vi "thermal measure Volt&SA.vi"(0 "meas_setting":T3={"measSetId"=6949, "measSetComments"="Orchid", "probeId"=141.0, "beamstyleIndex"=0, "txFrequencyHz"=3636400.0, "focusRangeCm"=8.0, "maxTxVoltageVolt"=100.0, "ceilTxVoltageVolt"=80.0, "profTxVoltageVolt"=62.0, "totalVoltagePt"=20, "numMeasVoltage"=12, "numTxElements"=118, "txpgWaveformStyle"=2, "numTxCycles"=4.0, "elevAperIndex"=0, "zStartDistCm"=1.5, "zMeasNum"=80, "IsTxAperModulationEn"=0, "DTxFreqIndex"=0, "VTxIndex"=0, "IsCPAEn"=0, "SysPulserSelA"=0, "TxPulseRleA"=""} {"zStartDistCm" format="%.2f"; "numTxCycles" format="%.1f"; "profTxVoltageVolt" format="%#_1g"; "ceilTxVoltageVolt" format="%.2f"; "maxTxVoltageVolt" format="%.2f"; "focusRangeCm" format="%.1f"; "txFrequencyHz" format="%.2f"}, 1 "PRF":dbl format="%.2f", 2 "CW":bool, 3 "measSetNum":i16, 4 "RoiLaterMin":dbl format="%.2f", 5 "TCP from Orchid in":refnum<k5>, 6 "RoiLateralSpan":dbl format="%.2f", 7 "Database":T4={"DB name"="zaop", "UID"="sel00752", "password"="rhkdwo7978"}, 8 "Measurement Type":enum32{"Volt", "SA"}(radio), 9 "tcp time out":dbl format="%.2f", 11 "voltage":dbl format="%.2f", 12 "Comment(SN)":string, 13 "Entire_element":u16, 14 "NumTxElement":i16) -> (10 "Command\nVerify":bool, 15 "Error(Volt & PRF)":bool)   [LabVIEW 2016]
uses:
  type def/Database.ctl
  type def/measSetting.ctl
  user/GrobaLimitVoltage.vi
  Thermal_type.vi
  <vilib>/Instr/_visa.llb/VISA Configure Serial Port (Instr).vi
  Instance          16 28Saved   thermal measure main .vi
  Instance          20 28Saved   thermal measure main .vi
panel:
  out "error out 4":errorcluster
  out "error out 3":errorcluster
  in  "취소 버튼":bool
  out "Measurement Time":enum32{"5min", "30min"}(radio)
  out "Voltage":dbl
  out "PRF":dbl
  out "right scanrange":dbl(slide) scale=0.0..30.1
  out "left scanrange":dbl(slide) max=3.0
  out "right aperture":u8(slide) scale=0.0..64.0
  out "left aperture":u8(slide) max=3
  out "경과시간(S)":string caption="경과 시간 텍스트"
  out "TempRise":dbl format="%.2f"
  out "Probe":dbl format="%.2f"
  out "Ambient":dbl format="%.2f"
  out "Waveform Chart":cluster{dbl, dbl}(graph)
  out "Actual PRF":dbl
  out "경과시간":dbl caption="경과 시간(초)" format="%#.1g"
  out "Ambient":dbl
  out "Transducer":dbl
  out "error out 2":errorcluster
  out "Input PRF":dbl format="%.2f"
  out "Current Voltage":dbl format="%.2f"
  out "Output Limit Voltage":i16
  out "Start Time":string="7/29/2002  5:00 PM"
  out "Finish Time":string="7/29/2002  5:00 PM"
  out "meas_temparature_output":T1 {"scanRange" format="%.2f"; "txpgWaveformStyle" format="%.2f"; "temperatureC" format="%.2f"; "pulseVoltage" format="%.2f"; "roomTempC" format="%.2f"; "probeId" format="%#.2f"}
  in  "stop 3":bool
  out "error out2":errorcluster
  in  "meas_temparature_result":T2={"probeId"=10.0, "comments"="4C1 WCS", "tempSSId"=2, "measDate"="", "measSetNum"=1, "roomTempC"=0.0, "pulseVoltage"=80.0, "temperatureC"=0.0, "numTxCycles"=3.0, "numTxElements"=22, "txFrequencyHz"=3636400, "elevAperIndex"=0, "isTxAperModulationEn"=0, "txpgWaveformStyle"=0.0, "pulseRepetRate"=610.0, "scanRange"=0.0, "tempSetId"=0, "IsSCW"=0, "VTxIndex"=0} {"temperatureC" format="%.2f"; "scanRange" format="%.2f"; "pulseRepetRate" format="%.6f"; "txpgWaveformStyle" format="%.3f"; "roomTempC" format="%.2f"; "numTxCycles" format="%#_1f"; "probeId" format="%#.2f"}
  in  "floating-point type conversion 2":string[][](table)=[["extended", "5", "12"], ["double", "5", "9"], ["single", "5", "5"]]
  out "Result":string
  in  "file path":path=path "C:/temp log data/TempResultData"
  out "error out":errorcluster
  # "Temperature Measurement"
  # "Cooling"
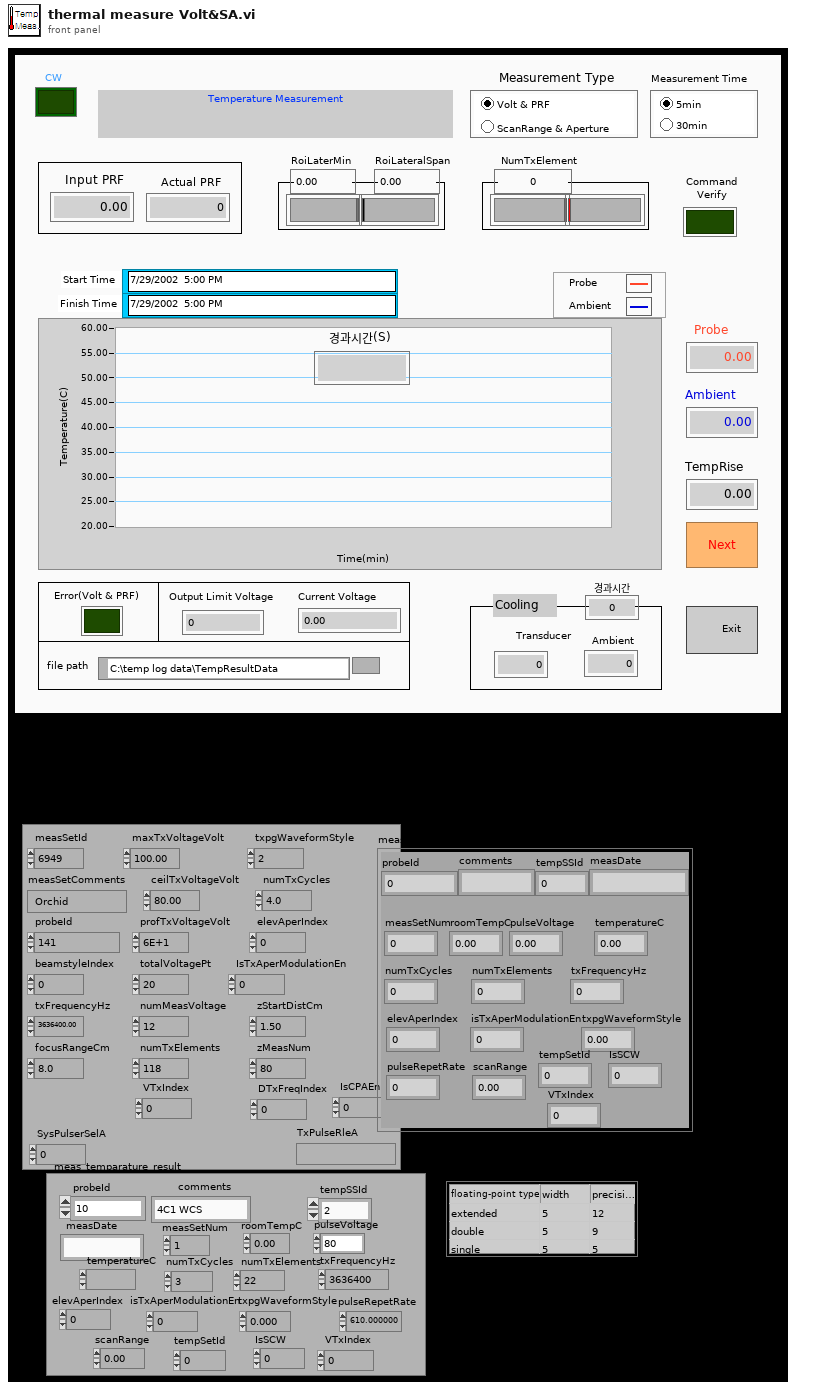
[diagram p1: front panel]
types:
  T1 = cluster{"probeId":sgl, "comments":string, "tempSSId":i16, "measDate":string, "measSetNum":i16, "roomTempC":sgl, "pulseVoltage":dbl, "temperatureC":ext, "numTxCycles":dbl, "numTxElements":i16, "txFrequencyHz":i32, "elevAperIndex":i16, "isTxAperModulationEn":i16, "txpgWaveformStyle":sgl, "pulseRepetRate":i32, "scanRange":dbl, "tempSetId":i16, "IsSCW":i16, "VTxIndex":i16}
  T2 = cluster{"probeId":sgl, "comments":string, "tempSSId":i16, "measDate":string, "measSetNum":i16, "roomTempC":sgl, "pulseVoltage":dbl, "temperatureC":ext, "numTxCycles":dbl, "numTxElements":i16, "txFrequencyHz":i32, "elevAperIndex":i16, "isTxAperModulationEn":i16, "txpgWaveformStyle":sgl, "pulseRepetRate":dbl, "scanRange":dbl, "tempSetId":i16, "IsSCW":i16, "VTxIndex":i8}
  T3 = typedef "measSetting.ctl" = cluster{"measSetId":i32, "measSetComments":string, "probeId":sgl, "beamstyleIndex":i16, "txFrequencyHz":sgl, "focusRangeCm":sgl, "maxTxVoltageVolt":sgl, "ceilTxVoltageVolt":sgl, "profTxVoltageVolt":dbl, "totalVoltagePt":i8, "numMeasVoltage":i8, "numTxElements":i16, "txpgWaveformStyle":i8, "numTxCycles":sgl, "elevAperIndex":i8, "zStartDistCm":sgl, "zMeasNum":i8, "IsTxAperModulationEn":i8, "DTxFreqIndex":i16, "VTxIndex":i8, "IsCPAEn":i16, "SysPulserSelA":i16, "TxPulseRleA":string}
  T4 = typedef "Database.ctl" = cluster{"DB name":string, "UID":string, "password":string}
  T5 = enum16{"open", "open or create", "create or replace", "create", "open (read only)"}
  T6 = cluster{"Output probe":dbl, "Output ambient":dbl}
  T7 = cluster{"status":bool, "code":i32, "text":string}
  T8 = typedef "Connection - Recordset reference.ctl" = cluster{"Connection":refnum<k7>, "Recordset":refnum<k7>}
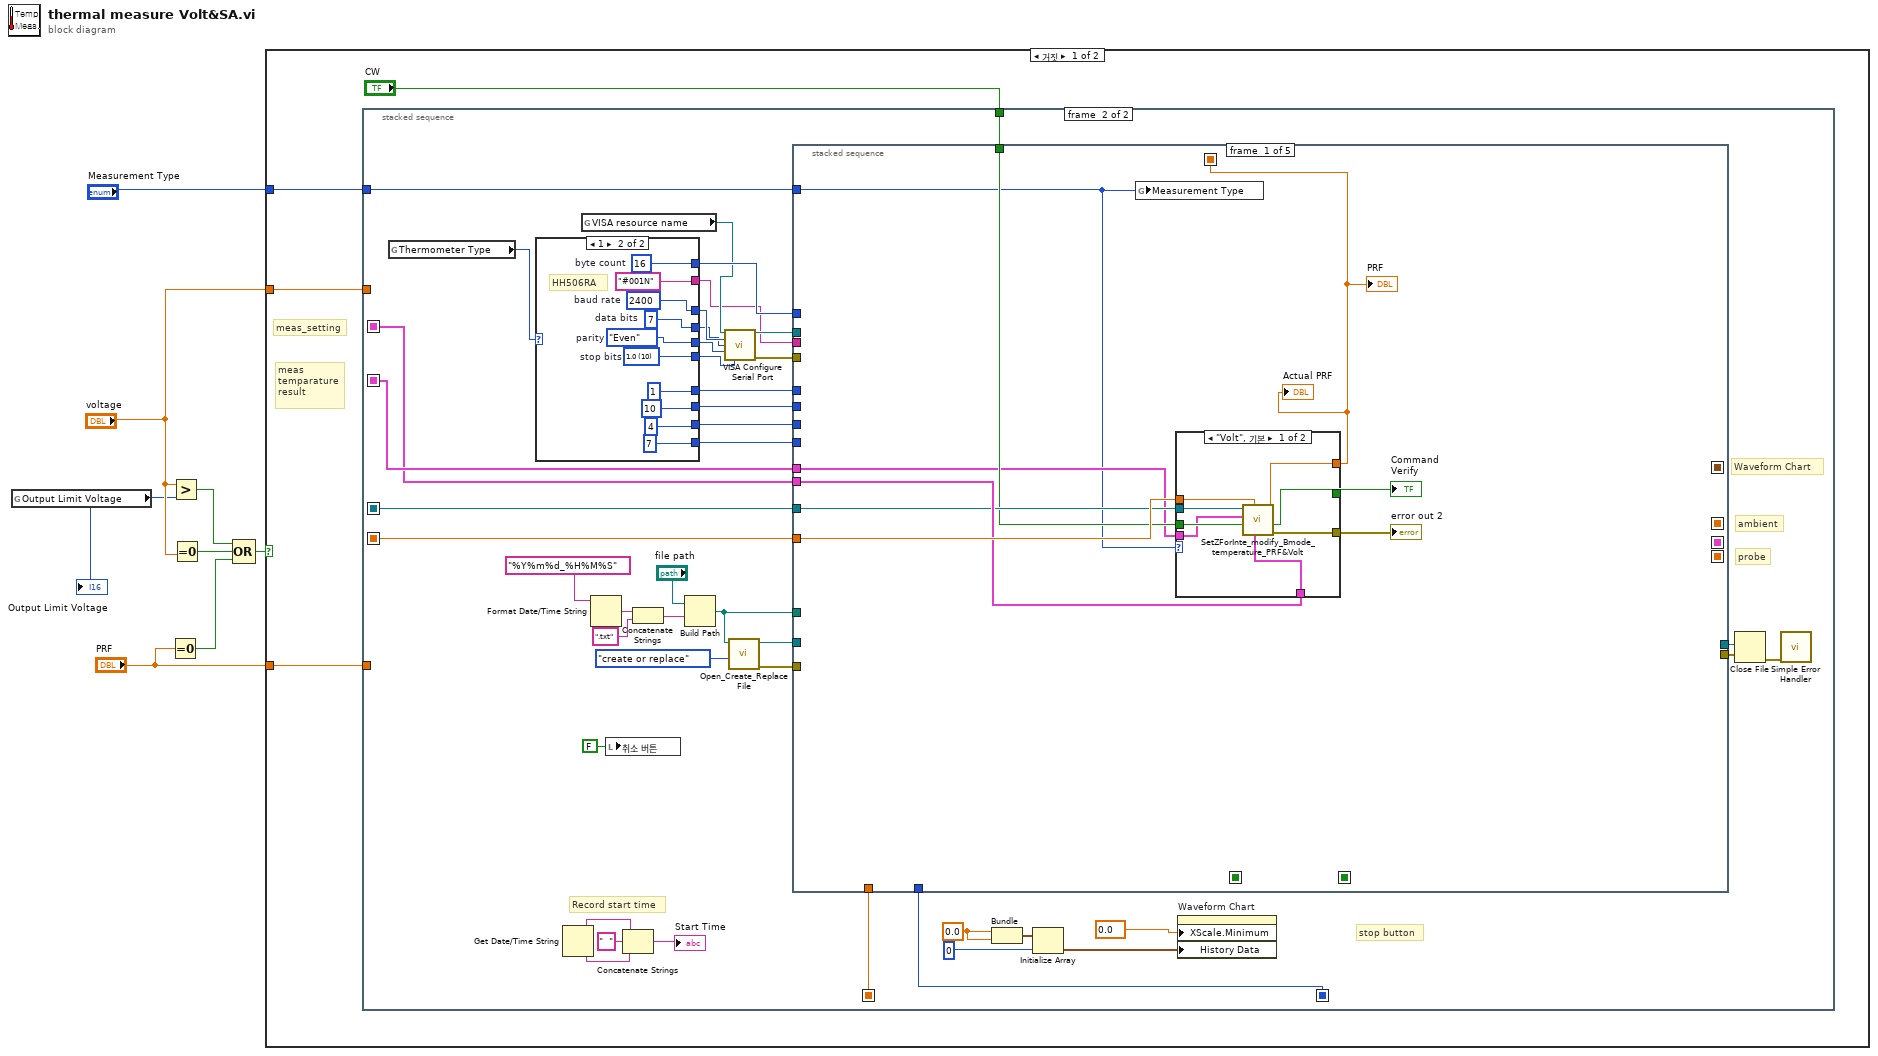
[diagram p0: block diagram]
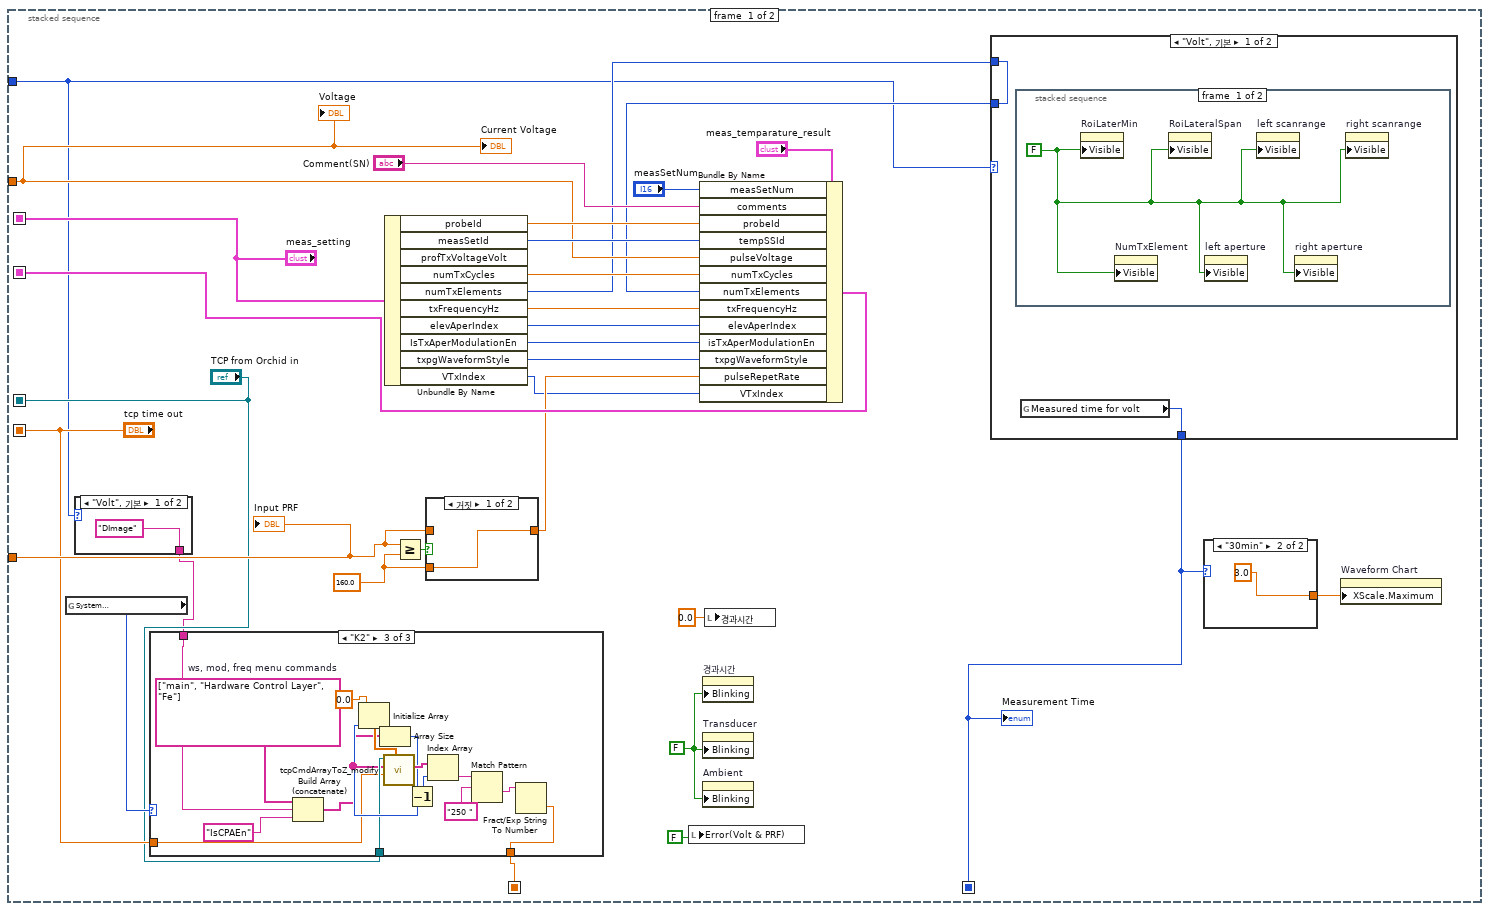
[diagram p2: hidden frame]
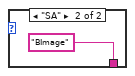
[diagram p3: hidden frame]
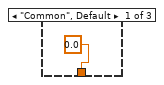
[diagram p4: hidden frame]
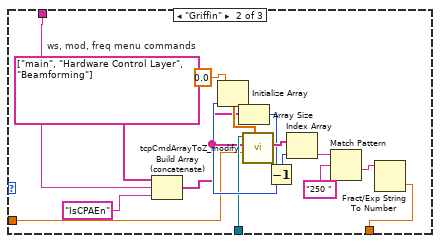
[diagram p5: hidden frame]
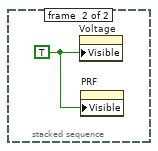
[diagram p7: hidden frame]
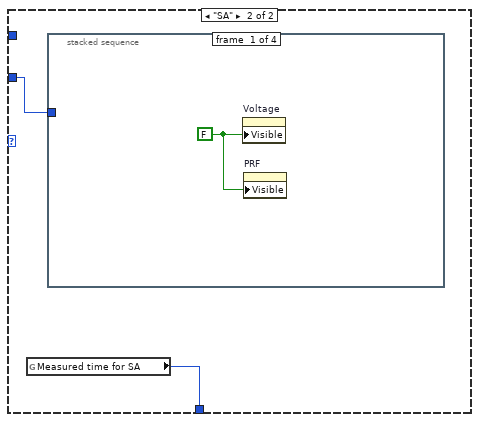
[diagram p8: hidden frame]
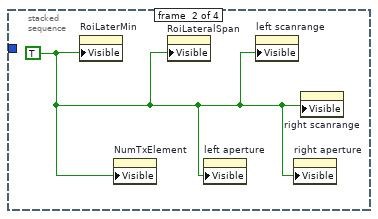
[diagram p9: hidden frame]
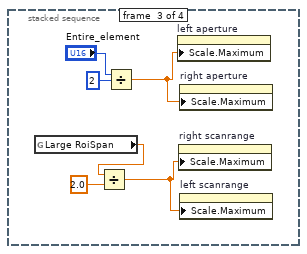
[diagram p10: hidden frame]
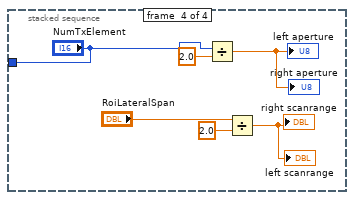
[diagram p11: hidden frame]
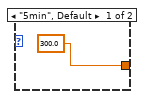
[diagram p12: hidden frame]
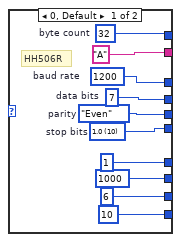
[diagram p13: hidden frame]
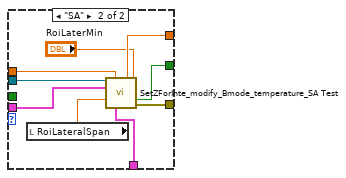
[diagram p14: hidden frame]
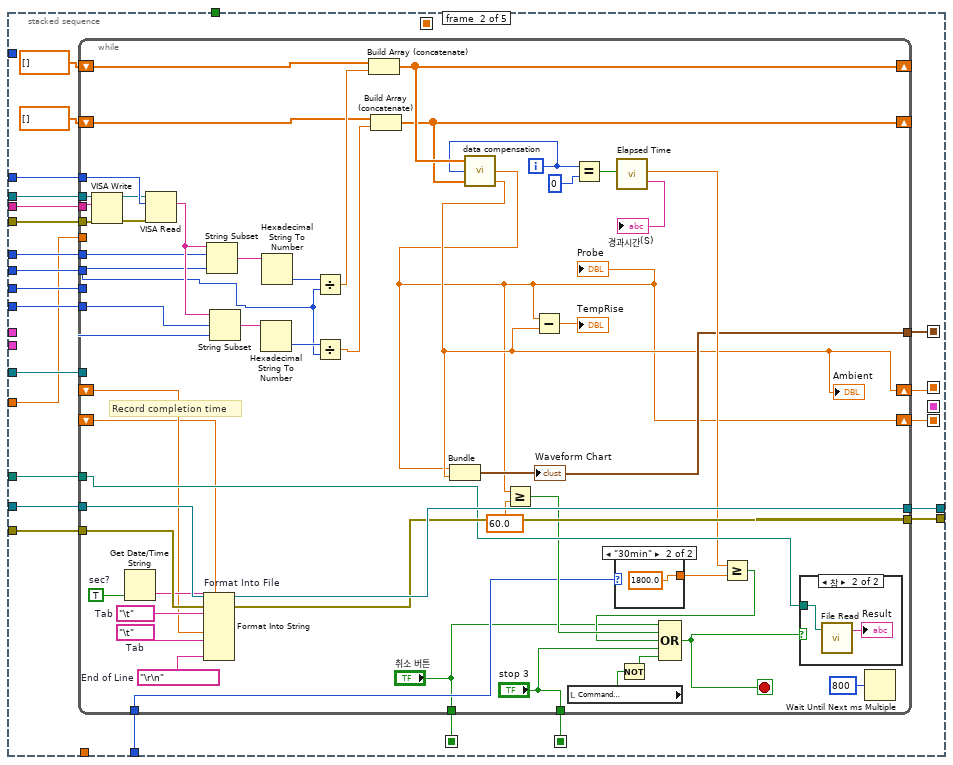
[diagram p15: hidden frame]
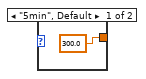
[diagram p16: hidden frame]
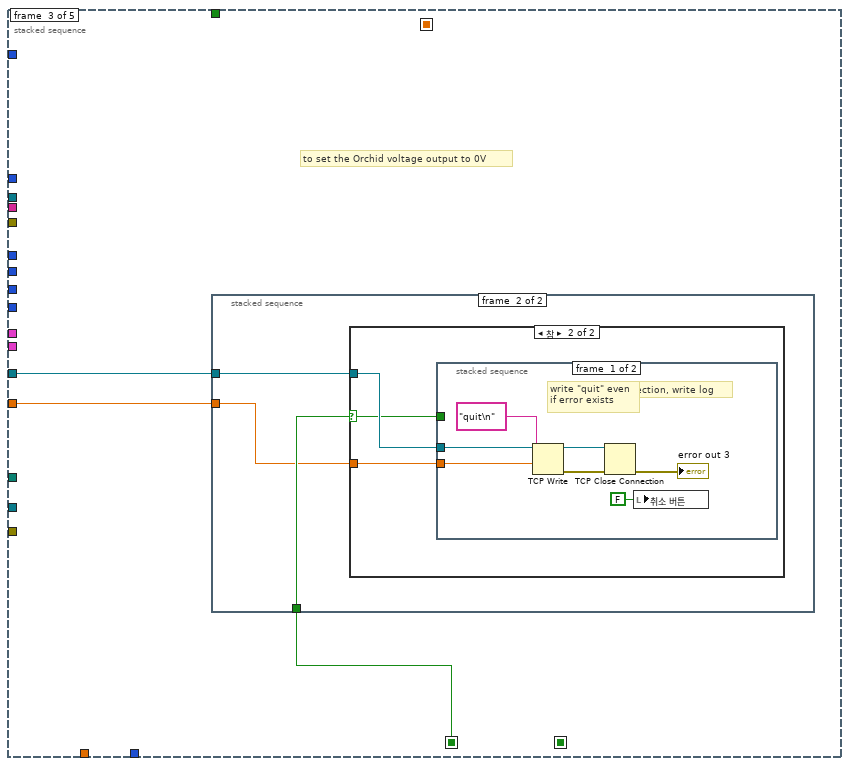
[diagram p18: hidden frame]
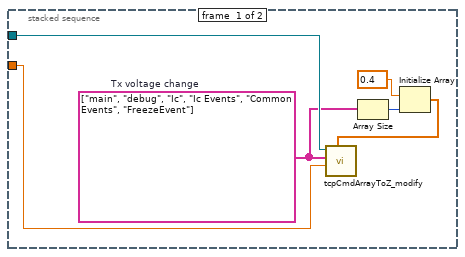
[diagram p19: hidden frame]
diagram:
  n1 = global read "GrobaLimitVoltage.vi" "Output Limit Voltage"() -> (w7:i16)
  "Output Limit Voltage" <- w7
  n2 = Equal To 0?(x="PRF") -> (x = 0?=w2:bool)
  n3 = Greater?(x="voltage", y=w7) -> (0:w6:bool)
  n4 = Equal To 0?(x="voltage") -> (x = 0?=w5:bool)
  n5 = Compound Arithmetic op=OR(w6, w5, w2) -> (w4:bool)
  n6 = case shown="거짓" w4 {
    tunnel: "voltage" -> [w12 _]
    tunnel: "PRF" -> [w11 _]
    tunnel: "Measurement Type" -> [w9 _]
    frame False {
      # "meas\ntemparature\nresult"
      # "meas_setting"
      n7 = stacked-sequence {
        seq-local: ["meas_setting" _] -> [_ w126]
        seq-local: [w34 _] -> [_ w133]
        seq-local: ["TCP from Orchid in" _] -> [_ w132]
        seq-local: ["tcp time out" _] -> [_ w131]
        seq-local: [w24 _] -> [_ w106]
        seq-local: [w16 _] -> [_ w101]
        tunnel: w12 -> [w32 _]
        tunnel: w11 -> [w21 _]
        tunnel: "CW" -> [_ w122]
        tunnel: w9 -> [w15 w103]
        frame #0 {
          w20 = 160.0 ("y")
          w30 = FALSE ("점멸")
          n8 = global read "Thermal_type.vi" "System \nSelection"() -> (w19:enum32{"Common", "Frosk", "Griffin", "K2"})
          n9 = case shown="\"Volt\", 기본" w15 {
            tunnel: ["DImage" "BImage"] -> w14
            frame "Volt", Default {
            }
            frame "SA" {
            }
          }
          n10 = case shown="\"K2\"" w19 {
            tunnel: [0.0 w54 w69] -> w16
            tunnel: "TCP from Orchid in" -> [_ w52 w67]
            tunnel: "tcp time out" -> [_ w51 w66]
            tunnel: w14 -> [_ w47 w62]
            frame "Common", Default {
            }
            frame "Griffin" {
              w50 = string[] ["main", "Hardware Control Layer", "Beamforming"]  # ws, mod, freq menu commands
              n11 = Build Array (concatenate)(w50, w47, "IsCPAEn") -> (w49:string[])
              n12 = Array Size(array=w49) -> (size(s)=w58:i32)
              n13 = Initialize Array(0.0 ("원소"), w58) -> (w60:dbl[])
              n14 = call "tcpCmdArrayToZ_modify.vi"("Delay (sec)"=w60, "Timeout (ms)"=w51, "Command array"=w49, "connection ID in"=w52) -> ("Receive array"=w59:string[])  [unwired: 3 in, 4 out]
              n15 = Decrement(x=w58) -> (x-1=w53:i32)
              n16 = Index Array(array=w59, index=w53) -> (element=w57:string)
              n17 = Match Pattern(string=w57, regular expression="250 " ("정규식")) -> (after substring=w56:string)  [unwired: 1 in, 3 out]
              n18 = Fract/Exp String To Number(string=w56) -> (number=w54:dbl)  [unwired: 3 in, 1 out]
            }
            frame "K2" {
              w65 = string[] ["main", "Hardware Control Layer", "Fe"]  # ws, mod, freq menu commands
              n19 = Build Array (concatenate)(w65, w62, "IsCPAEn") -> (w64:string[])
              n20 = Array Size(array=w64) -> (size(s)=w73:i32)
              n21 = Initialize Array(0.0 ("원소"), w73) -> (w75:dbl[])
              n22 = call "tcpCmdArrayToZ_modify.vi"("Delay (sec)"=w75, "Timeout (ms)"=w66, "Command array"=w64, "connection ID in"=w67) -> ("Receive array"=w74:string[])  [unwired: 3 in, 4 out]
              n23 = Decrement(x=w73) -> (x-1=w68:i32)
              n24 = Index Array(array=w74, index=w68) -> (element=w72:string)
              n25 = Match Pattern(string=w72, regular expression="250 " ("정규식")) -> (after substring=w71:string)  [unwired: 1 in, 3 out]
              n26 = Fract/Exp String To Number(string=w71) -> (number=w69:dbl)  [unwired: 3 in, 1 out]
            }
          }
          n27 = Unbundle By Name("meas_setting") -> ("probeId"=w41:sgl, "measSetId"=w40:i32, "numTxCycles"=w39:sgl, "numTxElements"=w27:i16, "txFrequencyHz"=w38:sgl, "elevAperIndex"=w37:i8, "IsTxAperModulationEn"=w36:i8, "txpgWaveformStyle"=w35:i8, "VTxIndex"=w13:i8)  [unwired: 1 out]
          n28 = Greater Or Equal?(x=w21, y=w20) -> (x >= y?=w23:bool)
          n29 = case shown="거짓" w23 {
            tunnel: [w77 w78] -> w22
            tunnel: w21 -> [_ w78]
            tunnel: w20 -> [w77 _]
            frame False {
            }
            frame True {
            }
          }
          n30 = local write "Error(Volt & PRF)"(FALSE) -> ()
          n31 = property on="경과시간" class="DigNum (엄격한)"("Blinking"=w30) -> ()  [unwired: 2 in, 2 out]
          n32 = property on="Transducer" class="DigNum (엄격한)"("Blinking"=w30) -> ()  [unwired: 2 in, 2 out]
          n33 = property on="Ambient" class="DigNum (엄격한)"("Blinking"=w30) -> ()  [unwired: 2 in, 2 out]
          n34 = local write "경과시간"(0.0 ("경과시간")) -> ()
          n35 = case shown="\"Volt\", 기본" w15 {
            tunnel: w27 -> [w80 _]
            tunnel: [w80 w84] -> w26
            tunnel: [w79 w83] -> w24
            frame "Volt", Default {
              n36 = stacked-sequence {
                frame #0 {
                  w81 = FALSE
                  n37 = property on="RoiLaterMin" class="DigNum (엄격한)"("Visible"=w81) -> ()  [unwired: 2 in, 2 out]
                  n38 = property on="NumTxElement" class="DigNum (엄격한)"("Visible"=w81) -> ()  [unwired: 2 in, 2 out]
                  n39 = property on="RoiLateralSpan" class="DigNum (엄격한)"("Visible"=w81) -> ()  [unwired: 2 in, 2 out]
                  n40 = property on="left aperture" class="Slide (엄격한)"("Visible"=w81) -> ()  [unwired: 2 in, 2 out]
                  n41 = property on="left scanrange" class="Slide (엄격한)"("Visible"=w81) -> ()  [unwired: 2 in, 2 out]
                  n42 = property on="right aperture" class="Slide (엄격한)"("Visible"=w81) -> ()  [unwired: 2 in, 2 out]
                  n43 = property on="right scanrange" class="Slide (엄격한)"("Visible"=w81) -> ()  [unwired: 2 in, 2 out]
                }
                frame #1 {
                  w82 = TRUE ("보이기")
                  n44 = property on="Voltage" class="DigNum (엄격한)"("Visible"=w82) -> ()  [unwired: 2 in, 2 out]
                  n45 = property on="PRF" class="DigNum (엄격한)"("Visible"=w82) -> ()  [unwired: 2 in, 2 out]
                }
              }
              n46 = global read "Thermal_type.vi" "Measured time for volt"() -> (w79:enum32{"5min", "30min"})
            }
            frame "SA" {
              n47 = global read "Thermal_type.vi" "Measured time for SA"() -> (w83:enum32{"5min", "30min"})
              n48 = stacked-sequence {
                tunnel: [_ _ _ "NumTxElement"] -> w84
                frame #0 {
                  w85 = FALSE ("보이기")
                  n49 = property on="Voltage" class="DigNum (엄격한)"("Visible"=w85) -> ()  [unwired: 2 in, 2 out]
                  n50 = property on="PRF" class="DigNum (엄격한)"("Visible"=w85) -> ()  [unwired: 2 in, 2 out]
                }
                frame #1 {
                  w86 = TRUE
                  n51 = property on="RoiLaterMin" class="DigNum (엄격한)"("Visible"=w86) -> ()  [unwired: 2 in, 2 out]
                  n52 = property on="NumTxElement" class="DigNum (엄격한)"("Visible"=w86) -> ()  [unwired: 2 in, 2 out]
                  n53 = property on="RoiLateralSpan" class="DigNum (엄격한)"("Visible"=w86) -> ()  [unwired: 2 in, 2 out]
                  n54 = property on="left aperture" class="Slide (엄격한)"("Visible"=w86) -> ()  [unwired: 2 in, 2 out]
                  n55 = property on="left scanrange" class="Slide (엄격한)"("Visible"=w86) -> ()  [unwired: 2 in, 2 out]
                  n56 = property on="right aperture" class="Slide (엄격한)"("Visible"=w86) -> ()  [unwired: 2 in, 2 out]
                  n57 = property on="right scanrange" class="Slide (엄격한)"("Visible"=w86) -> ()  [unwired: 2 in, 2 out]
                }
                frame #2 {
                  n58 = global read "Thermal_type.vi" "Large RoiSpan"() -> (w90:dbl)
                  n59 = Divide(x=w90, y=2.0) -> (x/y=w87:dbl)
                  n60 = Divide(x="Entire_element", y=u16 2) -> (x/y=w88:dbl)
                  n61 = property on="left aperture" class="Slide (엄격한)"("Scale.Maximum"=w88) -> ()  [unwired: 2 in, 2 out]
                  n62 = property on="right scanrange" class="Slide (엄격한)"("Scale.Maximum"=w87) -> ()  [unwired: 2 in, 2 out]
                  n63 = property on="right aperture" class="Slide (엄격한)"("Scale.Maximum"=w88) -> ()  [unwired: 2 in, 2 out]
                  n64 = property on="left scanrange" class="Slide (엄격한)"("Scale.Maximum"=w87) -> ()  [unwired: 2 in, 2 out]
                }
                frame #3 {
                  n65 = Divide(x="NumTxElement", y=2.0) -> (x/y=→"left aperture" →"right aperture":dbl)
                  n66 = Divide(x="RoiLateralSpan", y=2.0) -> (x/y=→"left scanrange" →"right scanrange":dbl)
                }
              }
            }
          }
          "Measurement Time" <- w24
          n67 = Bundle By Name(cluster="meas_temparature_result", "measSetNum"="measSetNum", "comments"="Comment(SN)", "probeId"=w41, "tempSSId"=w40, "pulseVoltage"=w32, "numTxCycles"=w39, "numTxElements"=w26, "txFrequencyHz"=w38, "elevAperIndex"=w37, "isTxAperModulationEn"=w36, "txpgWaveformStyle"=w35, "pulseRepetRate"=w22, "VTxIndex"=w13) -> (w34:T2)
          n68 = case shown="\"30min\"" w24 {
            tunnel: [300.0 ("y") 3.0 ("y")] -> w25
            frame "5min", Default {
            }
            frame "30min" {
            }
          }
          n69 = property on="Waveform Chart" class="WFChart (엄격한)"("XScale.Maximum"=w25) -> ()  [unwired: 2 in, 2 out]
          "Current Voltage" <- w32
          "Input PRF" <- w21
          "Voltage" <- w32
        }
        frame #1 {
          w107 = 0.0
          # "Record start time"
          # "Waveform Chart"
          # "ambient"
          # "probe"
          # "stop button"
          n70 = global read "Thermal_type.vi" "Thermometer Type"() -> (w121:u16)
          n71 = case shown="1" w121 {
            tunnel: [w154 w163] -> w119
            tunnel: [w153 w162] -> w118
            tunnel: [w152 w161] -> w117
            tunnel: ["A" ("write buffer (\"\")") "#001N" ("write buffer (\"\")")] -> w108
            tunnel: [w150 w160] -> w116
            tunnel: [10 ("offset (0)") 7 ("offset (0)")] -> w113
            tunnel: [6 ("length (rest)") 4 ("length (rest)")] -> w114
            tunnel: [u32 1000 ("y") u32 10 ("y")] -> w112
            tunnel: [1 ("offset (0)") 1 ("offset (0)")] -> w115
            tunnel: [w145 w155] -> w120
            frame 0, Default {
              w145 = u32 32  # byte count
              w150 = u16 10 items=["1.0"=10, "1.5"=15, "2.0"=20]  # stop bits
              w152 = enum16{"None", "Odd", "Even", "Mark", "Space"}."Even"  # parity
              w153 = u16 7  # data bits
              w154 = u32 1200  # baud rate
              # "HH506R"
            }
            frame 1 {
              w155 = u32 16  # byte count
              w160 = u16 10 items=["1.0"=10, "1.5"=15, "2.0"=20]  # stop bits
              w161 = enum16{"None", "Odd", "Even", "Mark", "Space"}."Even"  # parity
              w162 = u16 7  # data bits
              w163 = u32 2400  # baud rate
              # "HH506RA"
            }
          }
          n72 = Get Date/Time String() -> (date string=w129:string, time string=w127:string)  [unwired: 3 in]
          n73 = global read "Thermal_type.vi" "VISA resource name"() -> (w111:refnum<visa-resource-name>)
          n74 = Format Date/Time String(time format string (%c)="%Y%m%d_%H%M%S") -> (date/time string=w125:string)  [unwired: 2 in]
          n75 = local write "취소 버튼"(FALSE ("취소 버튼")) -> ()
          n76 = Concatenate Strings(w129, "  ", w127) -> (→"Start Time":string)
          n77 = Concatenate Strings(w125, ".txt" ("string")) -> (w134:string)
          n78 = Build Path(base path="file path", name or relative path=w134) -> (appended path=w135:path)
          n79 = call-poly "VISA Configure Serial Port"("VISA resource name"=w111, "baud rate (9600)"=w119, "data bits (8)"=w118, "parity (0:none)"=w117, "stop bits (10: 1 bit)"=w116) -> ("VISA resource name out"=w110:refnum<visa-resource-name>, "error out"=w109:errorcluster)  [unwired: 9 in]
          n80 = call <vilib>:"Open_Create_Replace File.vi"("function (open:0)"=T5."create or replace", "file path"=w135) -> ("error out"=w143:errorcluster, "refnum"=w144:refnum<file>)  [unwired: 6 in, 2 out]
          n81 = stacked-sequence {
            seq-local: [_ w208 _ _ _] -> [_ _ _ w304 _]
            seq-local: [_ w207 _ _ _] -> [_ _ _ w303 _]
            seq-local: [_ w206 _ _ _] -> [_ _ _ w300 _]
            seq-local: [_ _ _ w301 _] -> [_ _ _ _ w355]
            seq-local: [_ w205 _ _ _] -> [_ _ _ _ _]
            seq-local: [w166 _ _ _ _] -> [_ _ _ w297 _]
            seq-local: [_ w191 _ _ _] -> [_ _ w271 _ _]
            tunnel: w144 -> [_ w213 _ _ _]
            tunnel: w143 -> [_ w212 _ _ _]
            tunnel: [_ w211 _ _ _] -> w141
            tunnel: [_ w210 _ _ _] -> w139
            tunnel: w135 -> [_ w209 _ _ _]
            tunnel: w133 -> [w168 _ _ w302 _]
            tunnel: w132 -> [w171 w196 w273 w299 w365]
            tunnel: w131 -> [w173 w195 w272 w298 w364]
            tunnel: w126 -> [w172 _ _ _ w354]
            tunnel: w122 -> [w170 _ _ w296 _]
            tunnel: w120 -> [_ w204 _ _ w360]
            tunnel: w115 -> [_ w203 _ _ w363]
            tunnel: w114 -> [_ w202 _ _ w362]
            tunnel: w113 -> [_ w201 _ _ w356]
            tunnel: w112 -> [_ w200 _ _ w361]
            tunnel: w110 -> [_ w199 _ _ w359]
            tunnel: w109 -> [_ w198 _ _ w358]
            tunnel: w108 -> [_ w197 _ _ w357]
            tunnel: w106 -> [_ w194 _ _ _]
            tunnel: w103 -> [w165 _ _ w295 _]
            tunnel: w101 -> [_ _ _ w294 _]
            frame #0 {
              n82 = global write "Thermal_type.vi" "Measurement Type"(w165) -> ()
              n83 = case shown="\"Volt\", 기본" w165 {
                tunnel: w173 -> [w181 w182]
                tunnel: w172 -> [w180 w185]
                tunnel: w171 -> [w179 w188]
                tunnel: w170 -> [w178 _]
                tunnel: [w177 w184] -> w169
                tunnel: w168 -> [w176 w187]
                tunnel: [w175 w183] -> w167
                tunnel: [w174 w190] -> w166
                frame "Volt", Default {
                  n84 = call "SetZForInte_modify_Bmode_temperature_PRF&Volt.vi"("meas_setting"=w180, "timeout (ms)"=w181, "CW"=w178, "meas_temparature_Input"=w176, "TCP from Orchid in"=w179) -> ("error out"=w177:errorcluster, "veri_P/F"=w175:bool, "Actual PRF"=w174:dbl)  [unwired: 3 in, 1 out]
                }
                frame "SA" {
                  n85 = local read "RoiLateralSpan"() -> (w186:dbl)
                  n86 = call "SetZForInte_modify_Bmode_temperature_SA Test.vi"("TCP from Orchid in"=w188, "timeout (ms)"=w182, "RoiLaterMin"="RoiLaterMin", "meas_temparature_Input"=w187, "RoiLateralSpan"=w186, "meas_setting"=w185) -> ("Actual PRF"=w190:dbl, "veri_P/F"=w183:bool, "error out"=w184:errorcluster)  [unwired: 6 in, 1 out]
                }
              }
              "error out 2" <- w169
              "Command\nVerify" <- w167
              "Actual PRF" <- w166
              "PRF" <- w166
            }
            frame #1 {
              n87 = while {
                shift-right: [w216] -> w208
                shift-left: _ -> [w248]
                shift-right: [w215] -> w207
                shift-left: _ -> [w236]
                tunnel: w213 -> [w264]
                tunnel: w212 -> [w263]
                tunnel: [w262] -> w210
                tunnel: [w261] -> w211
                tunnel: w209 -> [w257]
                tunnel: ["stop 3"] -> w206
                tunnel: [w227] -> w205
                tunnel: w204 -> [w246]
                tunnel: w203 -> [w245]
                tunnel: w202 -> [w244]
                tunnel: w201 -> [w243]
                tunnel: w200 -> [w242]
                tunnel: w199 -> [w241]
                tunnel: w198 -> [w240]
                tunnel: w197 -> [w237]
                tunnel: w196 -> [_]
                tunnel: w195 -> [_]
                tunnel: w194 -> [w228]
                shift-right: [w220] -> _
                shift-left: dbl[] [] -> [w223]
                shift-right: [w218] -> _
                shift-left: dbl[] [] -> [w221]
                tunnel: ["취소 버튼"] -> w191
                i -> [w219]
                stop <- w255 stop-if-true
                w259 = "\t"  # Tab
                w260 = "\r\n"  # End of Line
                w265 = "\t"  # Tab
                w266 = TRUE  # sec?
                # "Record completion time"
                n88 = VISA Write(VISA resource name=w241, write buffer=w237, error in (no error)=w240) -> (VISA resource name out=w239:refnum<visa-resource-name>, error out=w238:errorcluster)  [unwired: 1 out]
                n89 = Get Date/Time String(want seconds? (F)=w266) -> (time string=w258:string)  [unwired: 2 in, 1 out]
                n90 = VISA Read(VISA resource name=w239, byte count=w246, error in (no error)=w238) -> (read buffer=w247:string)  [unwired: 3 out]
                n91 = Format Into String "Format Into File"(initial string=w264, error in=w263, w258, w265, w248, w259, w236, w260) -> (resulting string=w262:refnum<file>, error out=w261:errorcluster)  [unwired: 1 in]
                n92 = String Subset(string=w247, offset (0)=w245, length (rest)=w244) -> (substring=w252:string)
                n93 = String Subset(string=w247, offset (0)=w243, length (rest)=w244) -> (substring=w250:string)
                n94 = Hexadecimal String To Number(string=w250) -> (number=w249:u32)  [unwired: 2 in, 1 out]
                n95 = Hexadecimal String To Number(string=w252) -> (number=w251:u32)  [unwired: 2 in, 1 out]
                n96 = Divide(x=w251, y=w242) -> (x/y=w224:dbl)
                n97 = Divide(x=w249, y=w242) -> (x/y=w222:dbl)
                n98 = Build Array (concatenate)(w223, w224) -> (w220:dbl[])
                n99 = Build Array (concatenate)(w221, w222) -> (w218:dbl[])
                n100 = call "data compensation.vi"("Input ambient"=w218, "Index"=w219, "Input probe"=w220) -> ("Output ambient"=w216:dbl, "Output probe"=w215:dbl)  [unwired: 1 out]
                "Ambient" <- w216
                "Probe" <- w215
                n101 = Bundle("Output probe"=w215, "Output ambient"=w216) -> (w227:T6)  [unwired: 1 in]
                "Waveform Chart" <- w227
                n102 = Greater Or Equal?(x=w215, y=60.0) -> (x >= y?=w254:bool)
                n103 = Subtract(x=w215, y=w216) -> (x-y=→"TempRise":dbl)
                n104 = local read "Command\nVerify"() -> (w233:bool)
                n105 = Equal?(x=w219, y=0) -> (x = y?=w230:bool)
                n106 = case shown="\"30min\"" w228 {
                  tunnel: [300.0 ("y") 1800.0 ("y")] -> w229
                  frame "5min", Default {
                  }
                  frame "30min" {
                  }
                }
                n107 = call "Elapsed Time"("Reset"=w230) -> ("Elapsed Time (s)"=w235:dbl, "Elapsed Time Text"=→"경과시간(S)":string)  [unwired: 11 in, 6 out]
                n108 = Not(x=w233) -> (.not. x?=w232:bool)
                n109 = Greater Or Equal?(x=w235, y=w229) -> (x >= y?=w234:bool)
                n110 = Compound Arithmetic op=OR("취소 버튼", w254, w234, "stop 3", w232) -> (w255:bool)
                n111 = case shown="참" w255 {
                  tunnel: w257 -> [_ w269]
                  frame False {
                  }
                  frame True {
                    n112 = call "File Read.vi"("file path"=w269) -> ("data"=→"Result":string)  [unwired: 3 in]
                  }
                }
                n113 = Wait Until Next ms Multiple(millisecond multiple=u32 800 ("milliseconds to wait")) -> ()  [unwired: 1 out]
              }
            }
            frame #2 {
              # "to set the Orchid voltage output to 0V"
              n114 = stacked-sequence {
                tunnel: w273 -> [w279 w281]
                tunnel: w272 -> [w278 w280]
                tunnel: w271 -> [_ w282]
                frame #0 {
                  w275 = string[] ["main", "debug", "Ic", "Ic Events", "Common Events", "FreezeEvent"]  # Tx voltage change
                  n115 = Array Size(array=w275) -> (size(s)=w277:i32)
                  n116 = Initialize Array(0.4 ("element"), w277) -> (w274:dbl[])
                  n117 = call "tcpCmdArrayToZ_modify.vi"("Delay (sec)"=w274, "Timeout (ms)"=w278, "Command array"=w275, "connection ID in"=w279) -> ()  [unwired: 3 in, 5 out]
                }
                frame #1 {
                  n118 = case shown="참" w282 {
                    selector: w282 -> [_ w283]
                    tunnel: w281 -> [_ w285]
                    tunnel: w280 -> [_ w284]
                    frame False {
                    }
                    frame True {
                      n119 = stacked-sequence {
                        tunnel: w285 -> [w288 _]
                        tunnel: w284 -> [w287 _]
                        tunnel: w283 -> [_ w293]
                        frame #0 {
                          # "Close telnet connection, write log"
                          # "write \"quit\" even\nif error exists"
                          n120 = TCP Write(connection ID=w288, data in="quit\n", 9:w287) -> (connection ID out=w289:refnum<k5>, error out=w291:errorcluster)  [unwired: 1 in, 1 out]
                          n121 = TCP Close Connection(connection ID=w289, error in (no error)=w291) -> (error out=→"error out 3":errorcluster)  [unwired: 1 in, 1 out]
                          n122 = local write "취소 버튼"(FALSE ("취소 버튼")) -> ()
                        }
                        frame #1 {
                          n123 = Stop(stop? (T)=w293) -> ()
                        }
                      }
                    }
                  }
                }
              }
            }
            frame #3 {
              n124 = case shown="거짓" w300 {
                tunnel: w304 -> [w334 _]
                tunnel: w303 -> [w333 _]
                tunnel: w302 -> [w310 w353]
                tunnel: [w314 w353] -> w301
                tunnel: w299 -> [w318 _]
                tunnel: w298 -> [w317 _]
                tunnel: w297 -> [w312 _]
                tunnel: w296 -> [w311 _]
                tunnel: w295 -> [w309 _]
                tunnel: w294 -> [w305 _]
                frame False {
                  w308 = string[] ["main", "Hardware Control Layer", "Xp"]  # ScanRange
                  # "Record completion time"
                  n125 = Format Date/Time String(time format string (%c)="%Y-%m-%d %H:%M:%S" ("시간 포맷 문자열 (%c)")) -> (date/time string=w315:string)  [unwired: 2 in]
                  n126 = Get Date/Time String() -> (date string=w326:string, time string=w328:string)  [unwired: 3 in]
                  n127 = Concatenate Strings(w326, "  ", w328) -> (→"Finish Time":string)
                  n128 = case shown="참" w311 {
                    tunnel: [w350 w351] -> w313
                    tunnel: w312 -> [w350 _]
                    tunnel: w310 -> [_ w352]
                    frame False {
                    }
                    frame True {
                      n129 = Unbundle By Name(w352) -> ("txFrequencyHz"=w351:i32)
                    }
                  }
                  n130 = Unbundle By Name("Database") -> ("DB name"=w336:string, "UID"=w339:string, "password"=w338:string)
                  n131 = Format Into String(format string="UID=%s;\nPWD=%s;" ("Format String"), w339, w338) -> (resulting string=w337:string)  [unwired: 2 in, 1 out]
                  n132 = call <vilib>:"Connect.vi"("connection parameters"=w337, "data source name"=w336) -> ("error out"=w344:errorcluster, "Connection"=w345:refnum<k7>)  [unwired: 2 in]
                  n133 = case shown="\"Volt\", 기본" w309 {
                    tunnel: ["DImage" "BImage"] -> w307
                    frame "Volt", Default {
                    }
                    frame "SA" {
                    }
                  }
                  n134 = Build Array (concatenate)(w308, w307) -> (w306:string[])
                  n135 = call "tcpCmdArrayToZ_modify.vi"("Timeout (ms)"=w317, "Command array"=w306, "connection ID in"=w318) -> ("Receive array"=w324:string[])  [unwired: 4 in, 4 out]
                  n136 = Index Array(array=w324, index=3) -> (element=w322:string)
                  n137 = Match Pattern(string=w322, regular expression="ScanRangeCm\\t") -> (after substring=w320:string)  [unwired: 1 in, 3 out]
                  n138 = Fract/Exp String To Number(string=w320) -> (number=w319:dbl)  [unwired: 3 in, 1 out]
                  n139 = Bundle By Name(cluster=w310, "measDate"=w315, "roomTempC"=w334, "temperatureC"=w333, "scanRange"=w319, "pulseRepetRate"=w313, "IsSCW"=w305) -> (w314:T2)
                  n140 = call "MeasResSummToInsertZ JH.vi"("floating-point type conversion"="floating-point type conversion 2", "error in"=w344, "temperature"=w314, "connection reference"=w345) -> ("error out"=w343:T7, "insert sql statement"=w346:string, "connection reference"=w341:refnum<k7>)  [unwired: 3 in]
                  n141 = call <vilib>:"Execute SQL.vi"("error in (no error)"=w343, "SQL Statement"=w346, "Connection"=w341) -> ("error out"=w347:errorcluster, "reference"=w342:T8)
                  n142 = call <vilib>:"End SQL.vi"("error in (no error)"=w347, "reference"=w342) -> ("error out"=w329:errorcluster, "Connection"=w330:refnum<k7>)
                  n143 = call <vilib>:"Disconnect.vi"("error in (no error)"=w329, "connection"=w330) -> ("error out"=→"error out2":errorcluster)  [unwired: 1 in]
                }
                frame True {
                }
              }
            }
            frame #4 {
              n144 = stacked-sequence {
                seq-local: [w372 _] -> [_ w431]
                tunnel: [w383 _] -> w367
                tunnel: [w382 _] -> w366
                tunnel: w365 -> [_ w433]
                tunnel: w364 -> [_ w432]
                tunnel: w363 -> [w381 _]
                tunnel: w362 -> [w380 _]
                tunnel: w361 -> [w379 _]
                tunnel: w360 -> [w378 _]
                tunnel: w359 -> [w377 _]
                tunnel: w358 -> [w376 _]
                tunnel: w357 -> [w375 _]
                tunnel: w356 -> [w374 _]
                tunnel: w354 -> [_ _]
                frame #0 {
                  n145 = while {
                    tunnel: [w421] -> w383
                    tunnel: [w420] -> w382
                    tunnel: w381 -> [w419]
                    tunnel: w380 -> [w409]
                    tunnel: w379 -> [w407]
                    tunnel: w378 -> [w418]
                    tunnel: w377 -> [w417]
                    tunnel: w376 -> [w415]
                    tunnel: w375 -> [w413]
                    tunnel: w374 -> [w410]
                    shift-right: [w393] -> _
                    shift-left: dbl[] [] -> [w394]
                    tunnel: [w384] -> w372
                    stop <- w386 stop-if-true
                    w387 = TRUE ("점멸")
                    w400 = 1.0 ("y")
                    n146 = VISA Write(VISA resource name=w417, write buffer=w413, error in (no error)=w415) -> (VISA resource name out=w416:refnum<visa-resource-name>, error out=w414:errorcluster)  [unwired: 1 out]
                    n147 = VISA Read(VISA resource name=w416, byte count=w418, error in (no error)=w414) -> (VISA resource name out=w421:refnum<visa-resource-name>, read buffer=w411:string, error out=w420:errorcluster)  [unwired: 1 out]
                    n148 = String Subset(string=w411, offset (0)=w410, length (rest)=w409) -> (substring=w412:string)
                    n149 = String Subset(string=w411, offset (0)=w419, length (rest)=w409) -> (substring=w423:string)
                    n150 = property on="경과시간" class="DigNum (엄격한)"("Blinking"=w387) -> ()  [unwired: 2 in, 2 out]
                    n151 = property on="Transducer" class="DigNum (엄격한)"("Blinking"=w387) -> ()  [unwired: 2 in, 2 out]
                    n152 = property on="Ambient" class="DigNum (엄격한)"("Blinking"=w387) -> ()  [unwired: 2 in, 2 out]
                    n153 = Hexadecimal String To Number(string=w412) -> (number=w408:u32)  [unwired: 2 in, 1 out]
                    n154 = Hexadecimal String To Number(string=w423) -> (number=w422:u32)  [unwired: 2 in, 1 out]
                    n155 = Divide(x=w422, y=w407) -> (x/y=w395:dbl)
                    "Transducer" <- w395
                    n156 = Divide(x=w408, y=w407) -> (x/y=w396:dbl)
                    "Ambient" <- w396
                    n157 = local read "취소 버튼"() -> (w384:bool)
                    n158 = Build Array (concatenate)(w394, w395) -> (w393:dbl[])
                    n159 = Array Size(array=w393) -> (size(s)=w404:i32)
                    n160 = Subtract(x=w395, y=w396) -> (x-y=w406:dbl)
                    n161 = Decrement(x=w404) -> (x-1=w402:i32)
                    n162 = Absolute Value(x=w406) -> (abs(x)=w405:dbl)
                    n163 = Decrement(x=w402) -> (x-1=w403:i32)
                    n164 = Less Or Equal?(x=w405, y=w400) -> (x <= y?=w401:bool)
                    n165 = Index Array(array=w393, index=w402) -> (element=w391:dbl)
                    n166 = Index Array(array=w393, index=w403) -> (element=w392:dbl)
                    n167 = Subtract(x=w391, y=w392) -> (x-y=w390:dbl)
                    n168 = Divide(x=w400, y=2.0) -> (x/y=w398:dbl)
                    n169 = Absolute Value(x=w390) -> (abs(x)=w389:dbl)
                    n170 = Less Or Equal?(x=w389, y=w398) -> (x <= y?=w397:bool)
                    n171 = Compound Arithmetic op=AND(w397, w401) -> (w388:bool)
                    n172 = stacked-sequence {
                      seq-local: [w424 _] -> [_ w427]
                      tunnel: w388 -> [w425 _]
                      tunnel: [_ w430] -> w385
                      frame #0 {
                        n173 = case shown="참" w425 {
                          tunnel: [TRUE _] -> w424
                          frame False {
                          }
                          frame True {
                          }
                        }
                      }
                      frame #1 {
                        n174 = call "Elapsed Time2"("Reset"=w427) -> ("Elapsed Time (s)"=w429:dbl)  [unwired: 11 in, 7 out]
                        "경과시간" <- w429
                        n175 = Greater?(x=w429, y=60.0) -> (0:w430:bool)
                      }
                    }
                    n176 = Or(x=w385, y=w384) -> (x .or. y?=w386:bool)
                  }
                }
                frame #1 {
                  n177 = case shown="참" w431 {
                    tunnel: w433 -> [w440 w442]
                    tunnel: w432 -> [w439 w441]
                    tunnel: w431 -> [_ w443]
                    frame False {
                      w436 = string[] ["main", "debug", "Ic", "Ic Events", "Common Events", "FreezeEvent"]  # Tx voltage change
                      n178 = Array Size(array=w436) -> (size(s)=w438:i32)
                      n179 = Initialize Array(0.4 ("element"), w438) -> (w435:dbl[])
                      n180 = call "tcpCmdArrayToZ_modify.vi"("Delay (sec)"=w435, "Timeout (ms)"=w439, "Command array"=w436, "connection ID in"=w440) -> ()  [unwired: 3 in, 5 out]
                    }
                    frame True {
                      n181 = stacked-sequence {
                        tunnel: w442 -> [w446 _]
                        tunnel: w441 -> [w445 _]
                        tunnel: w443 -> [_ w451]
                        frame #0 {
                          # "Close telnet connection, write log"
                          # "write \"quit\" even\nif error exists"
                          n182 = TCP Write(connection ID=w446, data in="quit\n", 9:w445) -> (connection ID out=w447:refnum<k5>, error out=w449:errorcluster)  [unwired: 1 in, 1 out]
                          n183 = TCP Close Connection(connection ID=w447, error in (no error)=w449) -> (error out=→"error out 4":errorcluster)  [unwired: 1 in, 1 out]
                          n184 = local write "취소 버튼"(FALSE ("취소 버튼")) -> ()
                        }
                        frame #1 {
                          n185 = Stop(stop? (T)=w451) -> ()
                        }
                      }
                    }
                  }
                  n186 = local write "경과시간"(0.0 ("경과시간")) -> ()
                }
              }
              n187 = VISA Write(VISA resource name=w367, write buffer="B" ("write buffer (\"\")"), error in (no error)=w366) -> (VISA resource name out=w371:refnum<visa-resource-name>, error out=w370:errorcluster)  [unwired: 1 out]
              n188 = VISA Close(VISA resource name=w371, error in (no error)=w370) -> (error out=→"error out":errorcluster)
              "meas_temparature_output" <- w355
            }
          }
          n189 = Bundle(w107, w107) -> (w137:cluster{dbl, dbl})  [unwired: 1 in]
          n190 = Initialize Array(w137, 0) -> (w104:cluster{dbl, dbl}[])
          n191 = property on="Waveform Chart" class="WFChart (엄격한)"("XScale.Minimum"=0.0 ("X Scale.Range:Minimum"), "History Data"=w104) -> ()  [unwired: 2 in, 2 out]
          n192 = Close File(refnum=w139, error in=w141) -> (error out=w142:errorcluster)  [unwired: 1 out]
          n193 = call <vilib>:"Simple Error Handler.vi"("error in (no error)"=w142) -> ()  [unwired: 4 in, 5 out]
        }
      }
    }
    frame True {
      "Error(Volt & PRF)" <- TRUE
    }
  }
